vi "Backward Pass (RNN).vi"(0 "xs":dbl[][][](array[numeric])=[[[0.0], [1.0], [0.0]]], 5 "hs":dbl[][][](array[numeric])=[[[0.0], [0.0]], [[0.9959918876590693], [-0.9609924209716473]]] format="%_8f", 7 "ps":dbl[][][](array[numeric])=[[[0.2032853269546711], [0.10445737822381787], [0.6922572948215111]]] format="%_8f", 9 "targets":u64[](array[numeric])=[0], 11 "params":T2={"Wxh"=[[0.578129, 2.569937, -0.0219857], [-2.46959, 0.027262, 2.449614362]], "Whh"=[[-1.3996, 0.961745], [0.364566, -0.477064]], "bh"=[[0.535351], [-1.985987]], "Why"=[[-0.658616, 0.764692], [-1.7789986, 0.388036], [-0.130912, -0.333988]], "by"=[[-0.528417], [-0.44032], [-0.8844819]]} {"Wxh" format="%_8f"; "Whh" format="%_8f"; "bh" format="%_8f"; "Why" format="%_8f"; "by" format="%_8f"}) -> (6 "dParams_":T3={"dWxh"=[[0.0, 0.0019862373697962215, 0.0], [0.0, -0.06118825535684556, 0.0]], "dWhh"=[[0.0, 0.0], [0.0, 0.0]], "dbh"=[[0.0019862373697962215], [-0.06118825535684556]], "dWhy"=[[-0.7935213511320954, 0.7656367624734651], [0.10403870131705772, -0.10038274878765777], [0.6894826498150377, -0.6652540136858074]], "dby"=[[-0.796714673045329], [0.10445737822381787], [0.6922572948215111]]} {"dWxh" format="%_8f"; "dWhh" format="%_8f"; "dbh" format="%_8f"; "dWhy" format="%_8f"; "dby" format="%_8f"})   [LabVIEW 2014]
uses:
  <vilib>/Analysis/Matrix/Datatypes/RealMatrix.ctl
  <vilib>/Analysis/baseanly.llb/A x Vector.vi
  <vilib>/Analysis/Matrix/Numeric/Conversions/Array To Matrix - RA.vi
  <vilib>/Analysis/Matrix/Numeric/Add/Add - RM,RM.vi
  <vilib>/Analysis/Matrix/NI_Matrix.lvlib
  <vilib>/Analysis/NI_AALBase.lvlib
panel:
  in  "Tab Control":enum32{"Page 1", "Page 2", "Page 3", "Page 4"}(tab)
  out "t":u64
  out "t (reversed)":u64
  out "hs[t-1]":dbl[](array[numeric])
  out "hs[t]":dbl[](array[numeric])=[0.9959918876590693, -0.9609924209716473]
  out "dh":dbl[](array[numeric])=[0.2482747145029062, -0.7999137429267682] format="%_8f"
  out "dhraw":dbl[](array[numeric])=[0.0019862373697962215, -0.06118825535684556] format="%_8f"
  out "dhnext (in)":dbl[](array[numeric]) format="%_8f"
  out "dhnext (out)":dbl[](array[numeric])=[-0.02508709532519055, 0.031100967712772834] format="%_8f"
  out "dy":dbl[](array[numeric])=[-0.796714673045329, 0.10445737822381787, 0.6922572948215111] format="%_8f"
  out "input length":u64=1
  out "dby":T1=[[-0.796714673045329], [0.10445737822381787], [0.6922572948215111]] format="%_8f"
  out "dWxh":T1=[[0.0, 0.0019862373697962215, 0.0], [0.0, -0.06118825535684556, 0.0]] format="%_8f"
  out "dWhh":T1 format="%_8f"
  out "dbh":T1=[[0.0019862373697962215], [-0.06118825535684556]] format="%_8f"
  out "dWhy":T1=[[-0.7935213511320954, 0.7656367624734651], [0.10403870131705772, -0.10038274878765777], [0.6894826498150377, -0.6652540136858074]] format="%_8f"
  # "dParams (intermediate)"
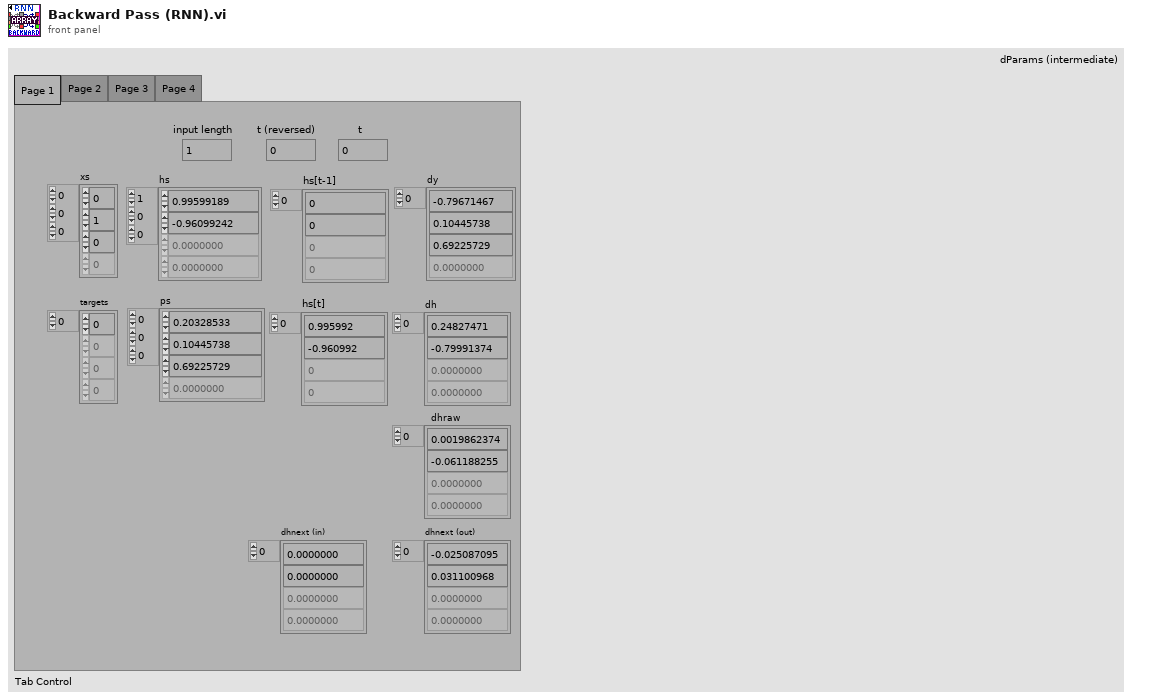
[diagram p1: front panel]
types:
  T1 = typedef "NI_Matrix.lvlib/RealMatrix.ctl" = dbl[][]
  T2 = cluster{"Wxh":T1, "Whh":T1, "bh":T1, "Why":T1, "by":T1}
  T3 = cluster{"dWxh":T1, "dWhh":T1, "dbh":T1, "dWhy":T1, "dby":T1}
  T4 = cluster{"Real Matrix":T1, "Real Matrix":T1, "Real Matrix (Column Vector)":T1, "Real Matrix":T1, "Real Matrix (Column Vector)":T1}
  T5 = cluster{"A + B":T1, "A + B":T1, "Real Matrix (Column Vector)":T1, "A + B":T1, "Real Matrix (Column Vector)":T1}
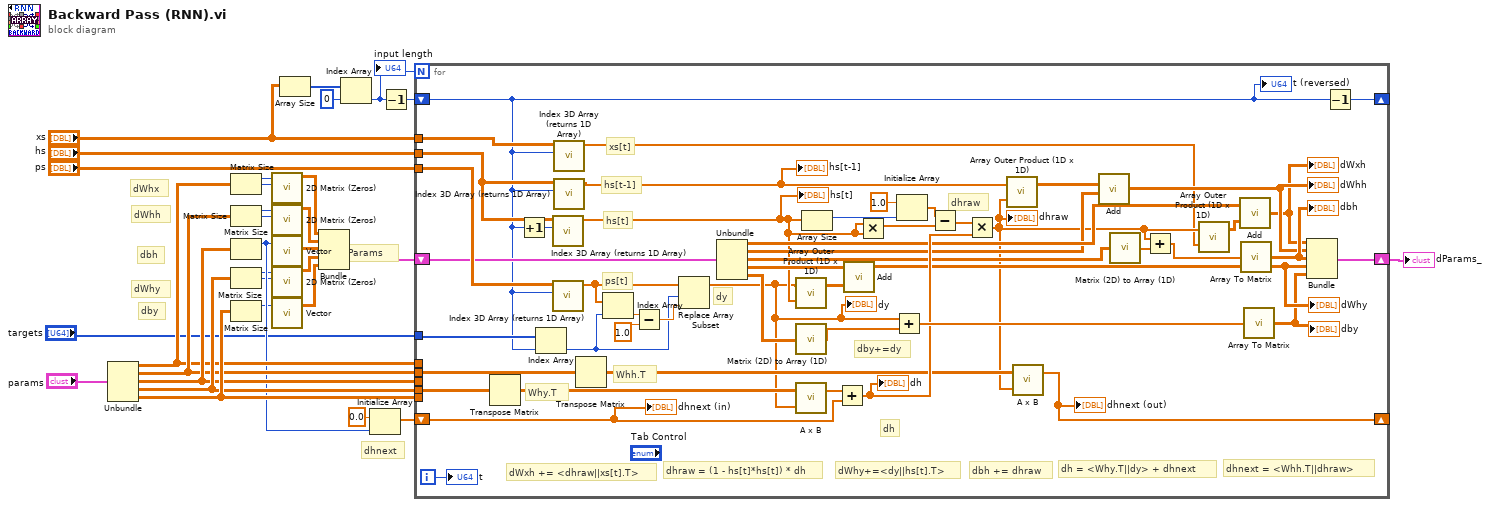
[diagram p0: block diagram]
diagram:
  # "dhnext"
  # "dWhx"
  # "dWhh"
  # "dby"
  # "dWhy"
  # "dbh"
  # "dParams"
  n1 = Unbundle("params") -> ("Wxh"=w23:T1, "Whh"=w24:T1, "bh"=w25:T1, "Why"=w26:T1, "by"=w27:T1)
  n2 = Matrix Size(0:w23) -> (1:w20:i32, 2:w11:i32)
  n3 = Matrix Size(0:w24) -> (1:w9:i32, 2:w10:i32)
  n4 = Matrix Size(0:w25) -> (1:w17:i32)  [unwired: 1 out]
  n5 = Matrix Size(0:w26) -> (1:w7:i32, 2:w8:i32)
  n6 = Matrix Size(0:w27) -> (1:w6:i32)  [unwired: 1 out]
  n7 = call "2D Matrix (Zeros).vi"("nCols (1)"=w11, "nRows"=w20) -> ("Real Matrix"=w16:T1)  [unwired: 9 in]
  n8 = call "2D Matrix (Zeros).vi"("nCols (1)"=w10, "nRows"=w9) -> ("Real Matrix"=w15:T1)  [unwired: 9 in]
  n9 = call "Vector.vi"("length"=w17) -> ("Real Matrix (Column Vector)"=w14:T1)  [unwired: 18 in]
  n10 = call "2D Matrix (Zeros).vi"("nCols (1)"=w8, "nRows"=w7) -> ("Real Matrix"=w13:T1)  [unwired: 9 in]
  n11 = call "Vector.vi"("length"=w6) -> ("Real Matrix (Column Vector)"=w12:T1)  [unwired: 18 in]
  n12 = Array Size(array="xs") -> (size(s)=w29:i32[])
  n13 = Bundle("Real Matrix"=w16, "Real Matrix"=w15, "Real Matrix (Column Vector)"=w14, "Real Matrix"=w13, "Real Matrix (Column Vector)"=w12) -> (w4:T4)  [unwired: 1 in]
  n14 = Index Array(array=w29, index=0) -> (element=w31:i32)
  "input length" <- w31
  n15 = Initialize Array(0.0 ("element"), w17) -> (w19:dbl[])
  n16 = Decrement(x=w31) -> (x-1=w5:i32)
  n17 = for {
    N: w31 -> [_]
    shift-right: [w55] -> w21
    shift-left: w4 -> [w70]
    tunnel: "xs" -> [w43]
    tunnel: "hs" -> [w42]
    tunnel: "ps" -> [w78]
    shift-right: [w80] -> _
    shift-left: w5 -> [w41]
    tunnel: "targets" -> [w79]
    shift-right: [w44] -> _
    shift-left: w19 -> [w45]
    tunnel: w26 -> [w54]
    tunnel: w24 -> [w53]
    tunnel: w23 -> [_]
    tunnel: w27 -> [_]
    tunnel: w25 -> [_]
    i -> [w81]
    # "dhnext = <Whh.T||dhraw>"
    # "dWxh += <dhraw||xs[t].T>"
    # "dbh += dhraw"
    # "dhraw = (1 - hs[t]*hs[t]) * dh"
    # "dh = <Why.T||dy> + dhnext"
    # "dWhy+=<dy||hs[t].T>"
    # "xs[t]"
    # "Whh.T"
    # "dy"
    # "dhraw"
    # "dh"
    # "Why.T"
    # "dby+=dy"
    # "hs[t-1]"
    # "hs[t]"
    # "ps[t]"
    n18 = Transpose Matrix(1:w54) -> (0:w67:T1)
    n19 = Increment(x=w41) -> (x+1=w40:i32)
    n20 = Index Array(array=w79, index=w41) -> (element=w73:u64)
    n21 = call "Index 3D Array (returns 1D Array).vi"("index"=w40, "3D array"=w42) -> ("1D array"=w33:dbl[])  [unwired: 9 in]
    "hs[t]" <- w33
    n22 = call "Index 3D Array (returns 1D Array).vi"("index"=w41, "3D array"=w78) -> ("1D array"=w75:dbl[])  [unwired: 9 in]
    n23 = call "Index 3D Array (returns 1D Array).vi"("index"=w41, "3D array"=w43) -> ("1D array"=w36:dbl[])  [unwired: 9 in]
    n24 = call "Index 3D Array (returns 1D Array).vi"("index"=w41, "3D array"=w42) -> ("1D array"=w38:dbl[])  [unwired: 9 in]
    "hs[t-1]" <- w38
    n25 = Transpose Matrix(1:w53) -> (0:w57:T1)
    n26 = Index Array(array=w75, index=w73) -> (element=w77:dbl)
    n27 = Subtract(x=w77, y=1.0) -> (x-y=w74:dbl)
    n28 = Replace Array Subset(array=w75, new element=w74, index=w73) -> (w32:dbl[])
    "dy" <- w32
    n29 = Unbundle(w70) -> ("Real Matrix"=w58:T1, "Real Matrix"=w47:T1, "Real Matrix (Column Vector)"=w59:T1, "Real Matrix"=w68:T1, "Real Matrix (Column Vector)"=w69:T1)
    n30 = call "Array Outer Product (1D x 1D).vi"("array a"=w32, "array b"=w33) -> ("a X b"=w34:dbl[][])  [unwired: 17 in]
    n31 = call "Matrix (2D) to Array (1D).vi"("Matrix (2D)"=w69) -> ("Array (1D)"=w71:dbl[])  [unwired: 4 in]
    n32 = call-poly <vilib>:"A x B.vi"("Vector"=w32, "A"=w67) -> ("A x Vector"=w66:dbl[])  [unwired: 1 out]
    n33 = Array Size(array=w33) -> (size(s)=w65:i32)
    n34 = Add ("Add.vi")(x=w66, y=w45) -> (x+y=w61:dbl[])
    "dh" <- w61
    n35 = call-poly <vilib>:"Add.vi"("Real Matrix B"=w34, "Real Matrix A"=w68) -> ("A + B"=w52:T1)
    "dWhy" <- w52
    n36 = Multiply(x=w33, y=w33) -> (x*y=w62:dbl[])
    n37 = Add(x=w32, y=w71) -> (x+y=w72:dbl[])
    n38 = Initialize Array(1.0 ("element"), w65) -> (w63:dbl[])
    n39 = Subtract(x=w63, y=w62) -> (x-y=w60:dbl[])
    n40 = Multiply(x=w60, y=w61) -> (x*y=w37:dbl[])
    "dhraw" <- w37
    n41 = call "Array Outer Product (1D x 1D).vi"("array a"=w38, "array b"=w37) -> ("a X b"=w39:dbl[][])  [unwired: 17 in]
    n42 = call-poly <vilib>:"A x B.vi"("Vector"=w37, "A"=w57) -> ("A x Vector"=w44:dbl[])  [unwired: 1 out]
    "dhnext (out)" <- w44
    n43 = call-poly <vilib>:"Add.vi"("Real Matrix B"=w47, "Real Matrix A"=w39) -> ("A + B"=w49:T1)
    "dWhh" <- w49
    n44 = call "Matrix (2D) to Array (1D).vi"("Matrix (2D)"=w59) -> ("Array (1D)"=w46:dbl[])  [unwired: 4 in]
    n45 = Add ("Add.vi")(x=w37, y=w46) -> (x+y=w56:dbl[])
    n46 = call "Array Outer Product (1D x 1D).vi"("array a"=w37, "array b"=w36) -> ("a X b"=w35:dbl[][])  [unwired: 17 in]
    n47 = call-poly <vilib>:"Add.vi"("Real Matrix B"=w35, "Real Matrix A"=w58) -> ("A + B"=w48:T1)
    "dWxh" <- w48
    n48 = call-poly <vilib>:"Array To Matrix.vi"("Real 1D Array"=w56) -> ("Real Matrix (Column Vector)"=w50:T1)
    "dbh" <- w50
    n49 = call-poly <vilib>:"Array To Matrix.vi"("Real 1D Array"=w72) -> ("Real Matrix (Column Vector)"=w51:T1)
    "dby" <- w51
    n50 = Bundle("A + B"=w48, "A + B"=w49, "Real Matrix (Column Vector)"=w50, "A + B"=w52, "Real Matrix (Column Vector)"=w51) -> (w55:T5)  [unwired: 1 in]
    n51 = Decrement(x=w41) -> (x-1=w80:i32)
    "t" <- w81
    "t (reversed)" <- w41
    "dhnext (in)" <- w45
  }
  "dParams_" <- w21
